vi "_Remote Set Voltages.vi"(4 "error in":errorcluster, 5 "Source/Gas":dbl[](array[numeric]), 6 "UserValues":dbl[](array[numeric]), 7 "VoltageType":T1=4 items=["Default", "Minimum", "Maximum", "Zero", "User"]) -> (0 "error out":errorcluster, 1 "Source/Gas Out":dbl[](array[numeric]), 2 "Voltages":dbl[](array[numeric]))   [LabVIEW 2018]
uses:
  Type/_Voltage Type.ctl
  Type/_RT Active Ch.ctl
  Type/_RT Command.ctl
  Type/_Model Family.ctl
  Configuration/_Global Configuration.vi
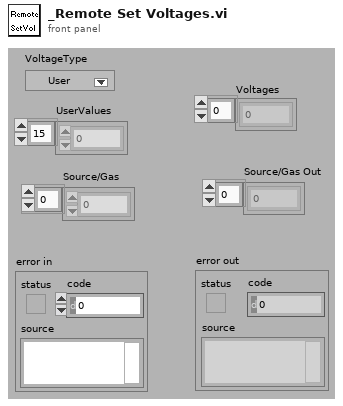
[diagram p1: front panel]
types:
  T1 = typedef "_Voltage Type.ctl" = u16
  T2 = typedef "_Model Family.ctl" = u16
  T3 = typedef "_RT Command.ctl" = enum16{"xml Start Run", "xml Start Actual Run", "xml Stop Run", "xml Runtime Update", "xml Get Status", "xml Get Table", "xml Set Table", "xml Get Configuration", "xml System Status", "xml Set LC Input Logic", "xml Get Data", "xml Get Info", "Start", "StartActualRun", "Stop", "Runtime Update", "Get Data", "Get Info", "Get Status", "Get Param", "Get Config", "Get Table", "Read ADC", "Set Oscillator", "Update Config", "Update Table", "Set All Pol", "Set Pol and DC", "Set Max Mass", "Toggle RP", "Toggle EL", "Set PIC", "Initialize Turbo", "Send Turbo Comm", "Close Turbo", "P1", "P2", "P3", "Send Serial", "Set LC Out", "Get LC In", "Read VAC", "Test Table", "Toggle Power", "Get Startup", "Set Startup", "Get ADC Table", "Set ADC Table", "Get Brief Status", "Get Detail Status", "Auxiliary Update", "Set CC Logics", "Test Channel", "Set CC Input Logics", "Ignore Error", "invalid"}
  T4 = typedef "_RT Active Ch.ctl" = cluster{"Start":i32, "Step":i32, "ChID":i32}
  T5 = typedef "_RT Configuration 2.ctl" = cluster{"Name":string, "Ch#":u8, "Min":dbl, "Max":dbl, "Def+":dbl, "Def-":dbl, "Offset":dbl, "Slope":dbl, "Type":u8, "Description":string, "SettleT":dbl}
  T6 = typedef "_RT Instrument 2.ctl" = cluster{"Table":T5[], "Instrument":string[]}
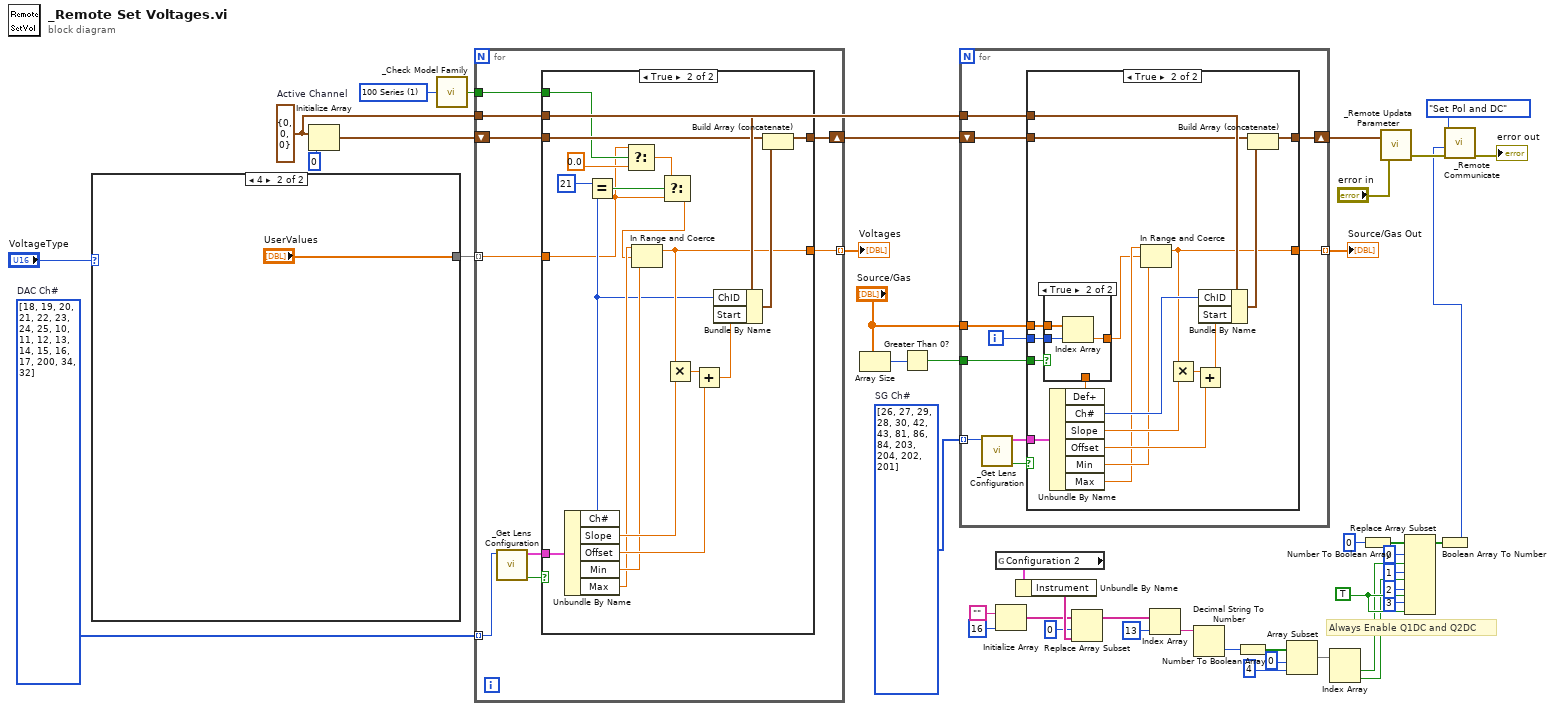
[diagram p0: block diagram]
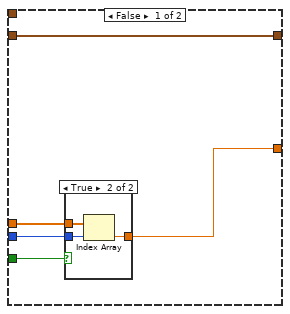
[diagram p2: hidden frame]
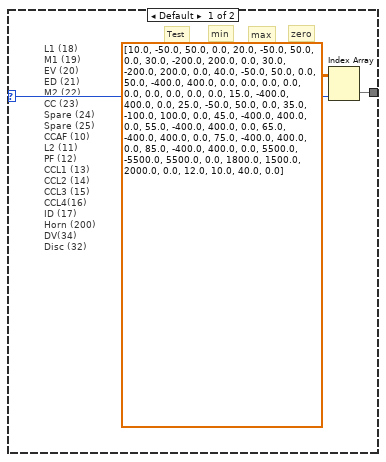
[diagram p6: hidden frame]
diagram:
  w2 = T2 1 items=["8080 Series", "100 Series", "200 Series", "300 Series", "Other Series"] ("Model Family (100)")
  w23 = TRUE
  w38 = u8[] [26, 27, 29, 28, 30, 42, 43, 81, 86, 84, 203, 204, 202, 201]  # SG Ch#
  w33 = T4 {"Start"=0, "Step"=0, "ChID"=0}  # Active Channel
  w43 = u8[] [18, 19, 20, 21, 22, 23, 24, 25, 10, 11, 12, 13, 14, 15, 16, 17, 200, 34, 32]  # DAC Ch#
  # "Always Enable Q1DC and Q2DC"
  n1 = case shown="4" "VoltageType" {
    selector: "VoltageType" -> [w47 _]
    tunnel: [w46 "UserValues"] -> w42
    frame Default {
      # "L1 (18)\nM1 (19)\nEV (20)\nED (21)\nM2 (22)\nCC (23)\nSpare (24)\nSpare (25)\nCCAF (10)\nL2 (11)\nPF (12)\nCCL1 (13)\nCCL2 (14)\nCCL3 (15)\nCCL4(16)\nID (17)\nHorn (200)\nDV(34)\nDisc (32)"
      # "zero"
      # "max"
      # "min"
      # "Test"
      n2 = Index Array(array=dbl[][] [[10.0, -50.0, 50.0, 0.0], [20.0, -50.0, 50.0, 0.0], [30.0, -200.0, 200.0, 0.0], [30.0, -200.0, 200.0, 0.0], [40.0, -50.0, 50.0, 0.0], [50.0, -400.0, 400.0, 0.0], [0.0, 0.0, 0.0, 0.0], [0.0, 0.0, 0.0, 0.0], [15.0, -400.0, 400.0, 0.0], [25.0, -50.0, 50.0, 0.0], [35.0, -100.0, 100.0, 0.0], [45.0, -400.0, 400.0, 0.0], [55.0, -400.0, 400.0, 0.0], [65.0, -400.0, 400.0, 0.0], [75.0, -400.0, 400.0, 0.0], [85.0, -400.0, 400.0, 0.0], [5500.0, -5500.0, 5500.0, 0.0], [1800.0, 1500.0, 2000.0, 0.0], [12.0, 10.0, 40.0, 0.0]], index (col)=w47) -> (element=w46:dbl[])  [unwired: 1 in]
    }
    frame 4 {
    }
  }
  n3 = Initialize Array(w33, 0 ("dimension size")) -> (w40:T4[])
  n4 = call "_Check Model Family.vi"("Model Family (100)"=w2) -> ("Yes"=w1:bool)
  n5 = for {
    tunnel: w43 -> [w51] mode=indexing
    tunnel: w42 -> [w53] mode=indexing
    shift-right: [w54] -> w34
    shift-left: w40 -> [w55]
    tunnel: w33 -> [w56]
    tunnel: [w52] -> w39 mode=indexing
    tunnel: w1 -> [w50]
    n6 = call "_Get Lens Configuration.vi"("Channel #"=w51) -> ("Found"=w58:bool, "Lens Configuration"=w57:T5)  [unwired: 1 in, 4 out]
    n7 = case shown="True" w58 {
      tunnel: w57 -> [_ w80]
      tunnel: w56 -> [_ w75]
      tunnel: w55 -> [w59 w74]
      tunnel: [w59 w72] -> w54
      tunnel: w53 -> [w60 w62]
      tunnel: [w60 w69] -> w52
      tunnel: w50 -> [_ w65]
      frame False {
      }
      frame True {
        n8 = Unbundle By Name(w80) -> ("Ch#"=w68:u8, "Slope"=w78:dbl, "Offset"=w77:dbl, "Min"=w71:dbl, "Max"=w70:dbl)
        n9 = Equal?(x=u8 21, y=w68) -> (x = y?=w64:bool)
        n10 = Select(t=w62, s=w65, f=0.0 ("t")) -> (s? t:f=w61:dbl)
        n11 = Select(t=w61, s=w64, f=w62) -> (s? t:f=w66:dbl)
        n12 = In Range and Coerce(upper limit=w70, x=w66, lower limit=w71) -> (coerced(x)=w69:dbl)  [unwired: 1 out]
        n13 = Multiply(x=w69, y=w78) -> (x*y=w79:dbl)
        n14 = Add(x=w79, y=w77) -> (x+y=w76:dbl)
        n15 = Bundle By Name(cluster=w75, "ChID"=w68, "Start"=w76) -> (w73:T4)
        n16 = Build Array (concatenate)(w74, w73) -> (w72:T4[])
      }
    }
  }
  "Voltages" <- w39
  n17 = Array Size(array="Source/Gas") -> (size(s)=w37:i32)
  n18 = Greater Than 0?(x=w37) -> (x > 0?=w36:bool)
  n19 = for {
    tunnel: w38 -> [w90] mode=indexing
    shift-right: [w85] -> w31
    shift-left: w34 -> [w86]
    tunnel: w33 -> [w87]
    tunnel: [w84] -> w32 mode=indexing
    tunnel: w36 -> [w83]
    tunnel: "Source/Gas" -> [w82]
    i -> [w81]
    n20 = call "_Get Lens Configuration.vi"("Channel #"=w90) -> ("Found"=w89:bool, "Lens Configuration"=w88:T5)  [unwired: 1 in, 4 out]
    n21 = case shown="True" w89 {
      tunnel: w88 -> [_ w116]
      tunnel: w87 -> [_ w111]
      tunnel: w86 -> [w95 w109]
      tunnel: [w95 w107] -> w85
      tunnel: [w91 w104] -> w84
      tunnel: w83 -> [w94 w103]
      tunnel: w82 -> [w92 w102]
      tunnel: w81 -> [w93 w101]
      frame False {
        n22 = case shown="True" w94 {
          tunnel: w92 -> [_ w98]
          tunnel: w93 -> [_ w97]
          tunnel: [_ w96] -> w91
          frame False {
          }
          frame True {
            n23 = Index Array(array=w98, index=w97) -> (element=w96:dbl)
          }
        }
      }
      frame True {
        n24 = Unbundle By Name(w116) -> ("Def+"=w99:dbl, "Ch#"=w110:u8, "Slope"=w114:dbl, "Offset"=w113:dbl, "Min"=w106:dbl, "Max"=w105:dbl)
        n25 = case shown="True" w103 {
          tunnel: w102 -> [_ w120]
          tunnel: w101 -> [_ w119]
          tunnel: [w117 w118] -> w100
          tunnel: w99 -> [w117 _]
          frame False {
          }
          frame True {
            n26 = Index Array(array=w120, index=w119) -> (element=w118:dbl)
          }
        }
        n27 = In Range and Coerce(upper limit=w105, x=w100, lower limit=w106) -> (coerced(x)=w104:dbl)  [unwired: 1 out]
        n28 = Multiply(x=w104, y=w114) -> (x*y=w115:dbl)
        n29 = Add(x=w115, y=w113) -> (x+y=w112:dbl)
        n30 = Bundle By Name(cluster=w111, "ChID"=w110, "Start"=w112) -> (w108:T4)
        n31 = Build Array (concatenate)(w109, w108) -> (w107:T4[])
      }
    }
  }
  "Source/Gas Out" <- w32
  n32 = global read "_Global Configuration.vi" "Configuration 2"() -> (w18:T6)
  n33 = Initialize Array("", 16 ("dimension size")) -> (w15:string[])
  n34 = Unbundle By Name(w18) -> ("Instrument"=w17:string[])
  n35 = Replace Array Subset(array=w15, new element=w17, index=0) -> (w6:string[])
  n36 = Index Array(array=w6, index=13) -> (element=w11:string)
  n37 = Decimal String To Number(string=w11) -> (number=w10:i32)  [unwired: 3 out]
  n38 = Number To Boolean Array(number=w10) -> (Boolean array=w9:bool[])
  n39 = Array Subset(array=w9, index=0, length=4) -> (w5:bool[])
  n40 = Index Array(array=w5) -> (element #1=w4:bool, element #2=w3:bool)  [unwired: 2 in]
  n41 = Number To Boolean Array(number=u16 0) -> (Boolean array=w25:bool[])
  n42 = call "_Remote Updata Parameter.vi"("error in"="error in", "Parameters"=w31) -> ("error out"=w22:errorcluster)
  n43 = Replace Array Subset(array=w25, new element #1=w4, index #1=0 ("index"), new element #2=w3, index #2=1 ("index"), new element #3=w23, index #3=2 ("index"), new element #4=w23, index #4=3 ("index")) -> (w30:bool[])
  n44 = Boolean Array To Number(Boolean array=w30) -> (number=w20:u16)
  n45 = call "_Remote Communicate.vi"("error in (no error)"=w22, "DC Param"=w20, "Command"=_RT_Command."Set Pol and DC") -> ("error out"=→"error out":errorcluster)  [unwired: 3 in, 3 out]
